vi "Simple Put File.vi"(0 "file uri":string, 1 "username":string, 2 "password":string, 7 "local file path":path, 11 "error in (no error)":errorcluster) -> (8 "local file path out":path, 15 "error out":errorcluster)   [LabVIEW 2020, in "NI_WebDAV.lvlib"]
doc: "Uploads a file or multiple files to a remote WebDAV server or target. You must manually select the polymorphic instance you want to use."
uses:
  <vilib>/WebDAVClient/NI_WebDAV.lvlib
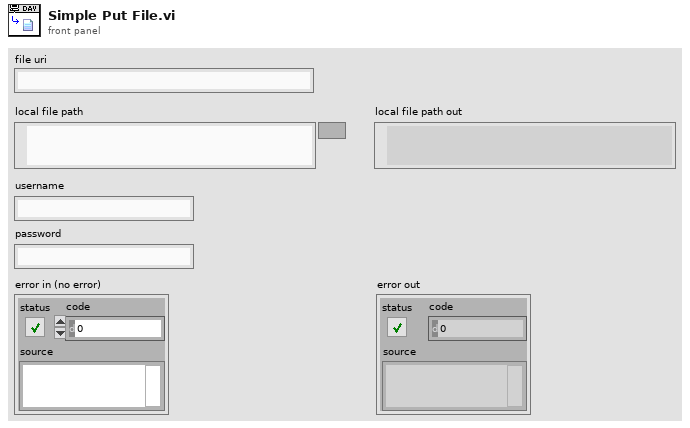
[diagram p1: front panel]
types:
  T1 = typedef "NI_WebDAV.lvlib/SessionHandle.ctl" = refnum<k1>
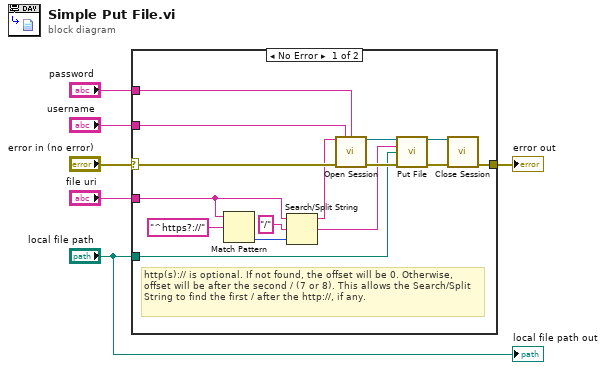
[diagram p0: block diagram]
diagram:
  n1 = case shown="No Error" "error in (no error)" {
    selector: "error in (no error)" -> [w21 w22]
    tunnel: "file uri" -> [w11 _]
    tunnel: "local file path" -> [w18 _]
    tunnel: "username" -> [w8 _]
    tunnel: "password" -> [w7 _]
    tunnel: [w15 w22] -> w1
    frame No Error {
      # "http(s):// is optional. If not found, the offset will be 0. Otherwise, offset will be after the second / (7 or 8). This allows the Search/Split String to find the first / after the http://, if any."
      n2 = Match Pattern(string=w11, regular expression="^https?://") -> (offset past match=w14:i32)  [unwired: 1 in, 3 out]
      n3 = Search/Split String(string=w11, search string/char (-)="/", offset (0)=w14) -> (substring before match=w10:string, match + rest of string=w9:string)  [unwired: 1 out]
      n4 = call <vilib>:"Open Session.vi"("host uri prefix"=w10, "username"=w8, "password"=w7, "error in (no error)"=w21) -> ("session handle out"=w19:T1, "error out"=w20:errorcluster)  [unwired: 10 in]
      n5 = call <vilib>:"Put File.vi"("session handle"=w19, "relative uri"=w9, "local file path"=w18, "error in (no error)"=w20) -> ("session handle out"=w16:T1, "error out"=w17:errorcluster)  [unwired: 9 in, 1 out]
      n6 = call <vilib>:"Close Session.vi"("session handle"=w16, "error in (no error)"=w17) -> ("error out"=w15:errorcluster)  [unwired: 13 in]
    }
    frame Error {
    }
  }
  "error out" <- w1
  "local file path out" <- "local file path"
